vi "From HW_Allrequest.vi"(5 "Plot window":string) -> (0 "Y name":string, 1 "Y signal":string, 2 "Ready?":bool, 3 "Y subarray":sgl[][](array[numeric]))   [LabVIEW 2021]
panel:
  out "Clone Name":string
  in  "Close windows":bool
  in  "Y data":string(combo)
  in  "Add":bool
  in  "Cancel":bool
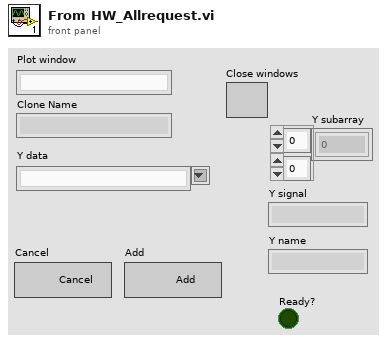
[diagram p1: front panel]
types:
  T1 = enum32{"Invalid", "Standard", "Closed", "Hidden", "Minimized", "Maximized"}
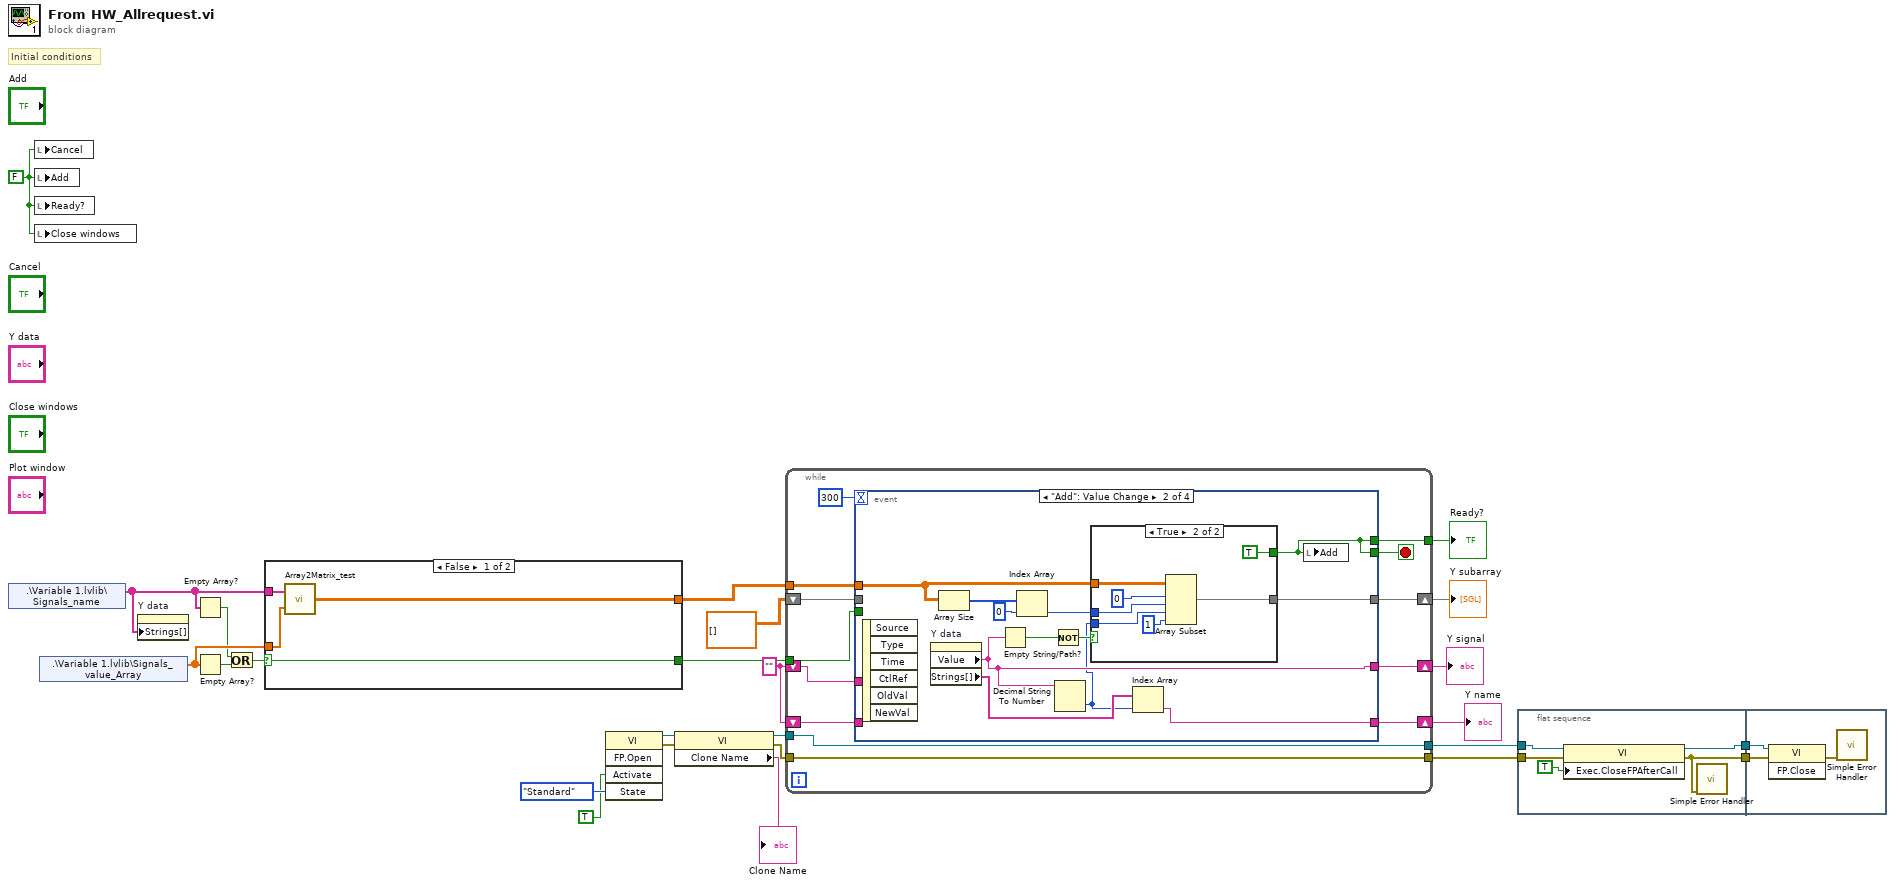
[diagram p0: block diagram]
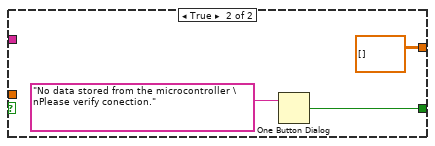
[diagram p2: hidden frame]
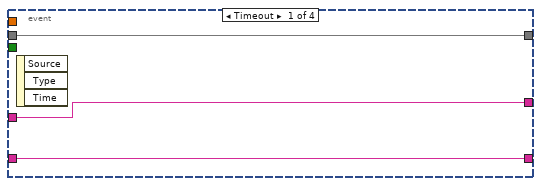
[diagram p3: hidden frame]
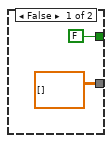
[diagram p4: hidden frame]
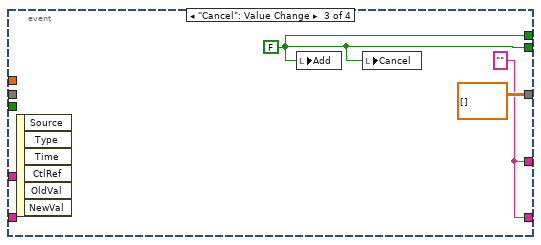
[diagram p5: hidden frame]
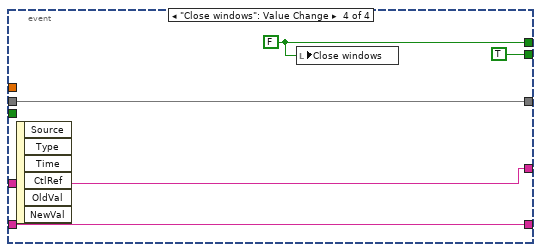
[diagram p6: hidden frame]
diagram:
  w2 = "" ("Value")
  w14 = FALSE
  # "Initial conditions"
  n1 = shared-variable ".\\Variable 1.lvlib\\Signals_name"() -> (w12:string[])  [unwired: 1 in, 1 out]
  n2 = local write "Cancel"(w14) -> ()
  n3 = local write "Add"(w14) -> ()
  n4 = local write "Ready?"(w14) -> ()
  n5 = local write "Close windows"(w14) -> ()
  n6 = shared-variable ".\\Variable 1.lvlib\\Signals_value_Array"() -> (w13:dbl[])  [unwired: 1 in, 1 out]
  n7 = property on="Y data" class="CmbBox"("Strings[]"=w12) -> ()  [unwired: 2 in, 2 out]
  n8 = Empty Array?(array=w12) -> (empty?=w10:bool)
  n9 = Empty Array?(array=w13) -> (empty?=w9:bool)
  n10 = Or(x=w10, y=w9) -> (x .or. y?=w11:bool)
  n11 = case shown="False" w11 {
    selector: w11 -> [w26 _]
    tunnel: w13 -> [w27 _]
    tunnel: [w29 sgl[][] [] ("Array2D")] -> w6
    tunnel: w12 -> [w28 _]
    tunnel: [w26 w30] -> w8
    frame False {
      n12 = call "Array2Matrix_test.vi"("Array"=w27, "Header"=w28) -> ("Array2D"=w29:sgl[][])
    }
    frame True {
      n13 = One Button Dialog(message="No data stored from the microcontroller \nPlease verify conection.") -> (true=w30:bool)  [unwired: 1 in]
    }
  }
  n14 = invoke on="Invoke Node" class="VI" method="FP.Open"("Activate"=TRUE ("Activate?"), "State"=T1."Standard") -> (reference out=w21:refnum<vi>, error out=w22:errorcluster)  [unwired: 3 in, 3 out]
  n15 = property on="Property Node" class="VI"(reference=w21, error in=w22) -> (reference out=w20:refnum<vi>, error out=w23:errorcluster, "Clone Name"=→"Clone Name":string)
  n16 = while {
    tunnel: [w45] -> w25
    tunnel: w23 -> [w43]
    tunnel: w20 -> [w44]
    tunnel: [w44] -> w18
    tunnel: [w43] -> w17
    tunnel: w8 -> [w38]
    tunnel: w6 -> [w36]
    shift-right: [w41] -> w7
    shift-left: sgl[][] [] ("all rows") -> [w42]
    shift-right: [w40] -> w3
    shift-left: w2 -> [w35]
    shift-right: [w34] -> w4
    shift-left: w2 -> [w33]
    stop <- w37 stop-if-true
    n17 = event shown="[1] \"Add\": Value Change" {
      selector: _ -> [_ _ _ _]
      dyn-events: _ -> [_ _ _ _]
      timeout: 300 -> [_ _ _ _]
      tunnel: [_ w60 w71 TRUE] -> w37
      tunnel: [_ w60 w71 w76] -> w45
      tunnel: w42 -> [w48 _ _ w75]
      tunnel: [w48 w59 sgl[][] [] ("all rows") w75] -> w41
      tunnel: [w47 w52 w70 w74] -> w40
      tunnel: w38 -> [_ _ _ _]
      tunnel: w36 -> [_ w53 _ _]
      tunnel: w35 -> [w47 _ _ w74]
      tunnel: [w46 w49 w70 w73] -> w34
      tunnel: w33 -> [w46 _ _ w73]
      event Timeout {
        n18 = event-data() -> ()  [unwired: 1 in, 3 out]
      }
      event "Add": Value Change {
        n19 = event-data() -> ()  [unwired: 1 in, 6 out]
        n20 = property on="Y data" class="CmbBox"() -> ("Value"=w52:string, "Strings[]"=w51:string[])  [unwired: 2 in, 2 out]
        n21 = Array Size(array=w53) -> (size(s)=w58:i32[])
        n22 = Empty String/Path?(string/path=w52) -> (empty?=w54:bool)
        n23 = Index Array(array=w58, index=0) -> (element=w56:i32)
        n24 = Not(x=w54) -> (.not. x?=w55:bool)
        n25 = Decimal String To Number(string=w52) -> (number=w50:i32)  [unwired: 2 in, 1 out]
        n26 = case shown="True" w55 {
          tunnel: [FALSE TRUE] -> w60
          tunnel: w53 -> [_ w65]
          tunnel: w50 -> [_ w68]
          tunnel: [sgl[][] [] w66] -> w59
          tunnel: w56 -> [_ w64]
          frame False {
          }
          frame True {
            n27 = Array Subset(array=w65, index (row)=0 ("index"), length (row)=w64, index (col)=w68, length (col)=1 ("length")) -> (w66:sgl[][])
          }
        }
        n28 = Index Array(array=w51, index=w50) -> (element=w49:string)
        n29 = local write "Add"(w60) -> ()
      }
      event "Cancel": Value Change {
        w70 = "" ("Value")
        w71 = FALSE
        n30 = event-data() -> ()  [unwired: 1 in, 6 out]
        n31 = local write "Add"(w71) -> ()
        n32 = local write "Cancel"(w71) -> ()
      }
      event "Close windows": Value Change {
        w76 = FALSE
        n33 = event-data() -> ()  [unwired: 1 in, 6 out]
        n34 = local write "Close windows"(w76) -> ()
      }
    }
  }
  "Ready?" <- w25
  "Y subarray" <- w7
  "Y name" <- w4
  "Y signal" <- w3
  n35 = flat-sequence {
    tunnel: w18 -> [w82]
    tunnel: w17 -> [w81]
    tunnel: [w79] -> w16
    tunnel: [w78] -> w15
    tunnel: w16 -> [w84]
    tunnel: w15 -> [w83]
    frame #0 {
      n36 = property class="VI"(reference=w82, error in=w81, "Exec.CloseFPAfterCall"=TRUE ("Activate?")) -> (reference out=w79:refnum<vi>, error out=w78:errorcluster)
      n37 = call <vilib>:"Simple Error Handler.vi"("error in (no error)"=w78) -> ()  [unwired: 4 in, 5 out]
    }
    frame #1 {
      n38 = invoke class="VI" method="FP.Close"(reference=w84, error in=w83) -> (error out=w85:errorcluster)  [unwired: 1 in, 2 out]
      n39 = call <vilib>:"Simple Error Handler.vi"("error in (no error)"=w85) -> ()  [unwired: 4 in, 5 out]
    }
  }
